vi "set_refdac.vi"(0 "TSM context":T2, 5 "Config PVS":T1 {"VREFN" format="%#_13g"; "AVOUT" format="%#_13g"; "VREFP" format="%#_13g"; "Read/Write" items=["Write", "Read"]}, 11 "Error In":errorcluster) -> (4 "TSM context Out":T2, 15 "Error Out":errorcluster)   [LabVIEW 2019]
doc: "This VI set the output voltage of Precision Voltage Source (PVS)"
uses:
  <vilib>/NI_TestStand_SemiconductorModule/NI_TestStand_Semiconductor_Module.lvlibp/PinMap/General/SemiconductorModuleContext.ctl
  typedefs/set_refdac_param.ctl
  <instrlib>/niDigital/niDigital.llb/niDigital Selected Function.ctl
  <instrlib>/niDigital/niDigital.llb/niDigital Write Static Pin State.ctl
  <instrlib>/niDigital/niDigital.llb/niDigital Data Mapping.ctl
  <instrlib>/niDigital/niDigital.llb/niDigital Bit Order.ctl
  Instrument Control/Digital/SSC Digital/Configuration/SSC Digital Select Function.vi
  Instrument Control/Digital/SSC Digital/Static/SSC Digital Write Static.vi
  <instrlib>/niDigital/niDigital.llb/niDigital Create Source Waveform (Serial).vi
  <instrlib>/niDigital/niDigital.llb/niDigital Write Source Waveform (Broadcast U32).vi
  <instrlib>/niDigital/niDigital.llb/niDigital Burst Pattern (Pass Fail).vi
  <vilib>/NI_TestStand_SemiconductorModule/NI_TestStand_Semiconductor_Module.lvlibp/PinMap/Digital Pattern/PinsToNIDigitalPatternSessions.vi
  <vilib>/NI_TestStand_SemiconductorModule/NI_TestStand_Semiconductor_Module.lvlibp
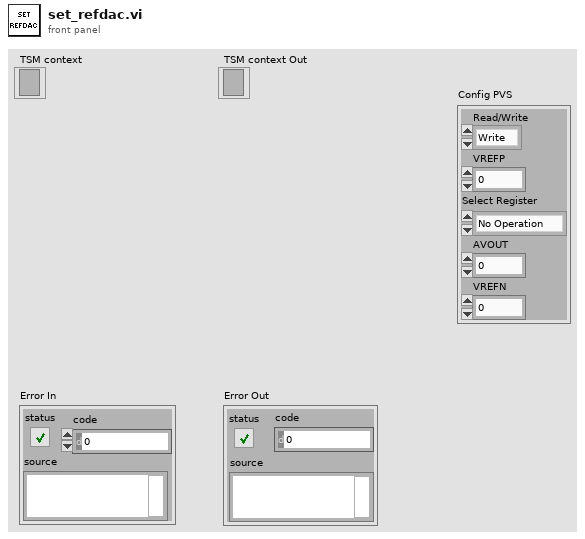
[diagram p1: front panel]
types:
  T1 = typedef "set_refdac_param.ctl" = cluster{"Read/Write":u16, "VREFP":dbl, "Select Register":enum16{"No Operation", "DAC Register", "Control Register", "Clearcode Register", "Software Control Register"}, "AVOUT ":dbl, "VREFN":dbl}
  T2 = typedef "NI_TestStand_Semiconductor_Module.lvlibp/SemiconductorModuleContext.ctl" = refnum<k7>
  T3 = enum16{"No Operation", "DAC Register", "Control Register", "Clearcode Register", "Software Control Register"}
  T4 = typedef "niDigital Bit Order.ctl" = i32
  T5 = typedef "niDigital Data Mapping.ctl" = i32
  T6 = typedef "niDigital Write Static Pin State.ctl" = u8
  T7 = typedef "niDigital Selected Function.ctl" = i32
  T8 = typedef "TSM SSC Digital.ctl" = cluster{"Pin Query Context":refnum<class "DigitalPatternPinQueryContext.lvclass">, "SSC":T9[], "Site Numbers":i32[], "Pins":tag[]}
  T9 = typedef "SSC Digital.ctl" = cluster{"Session":refnum<k15>, "Channel List":string, "Site List":string}
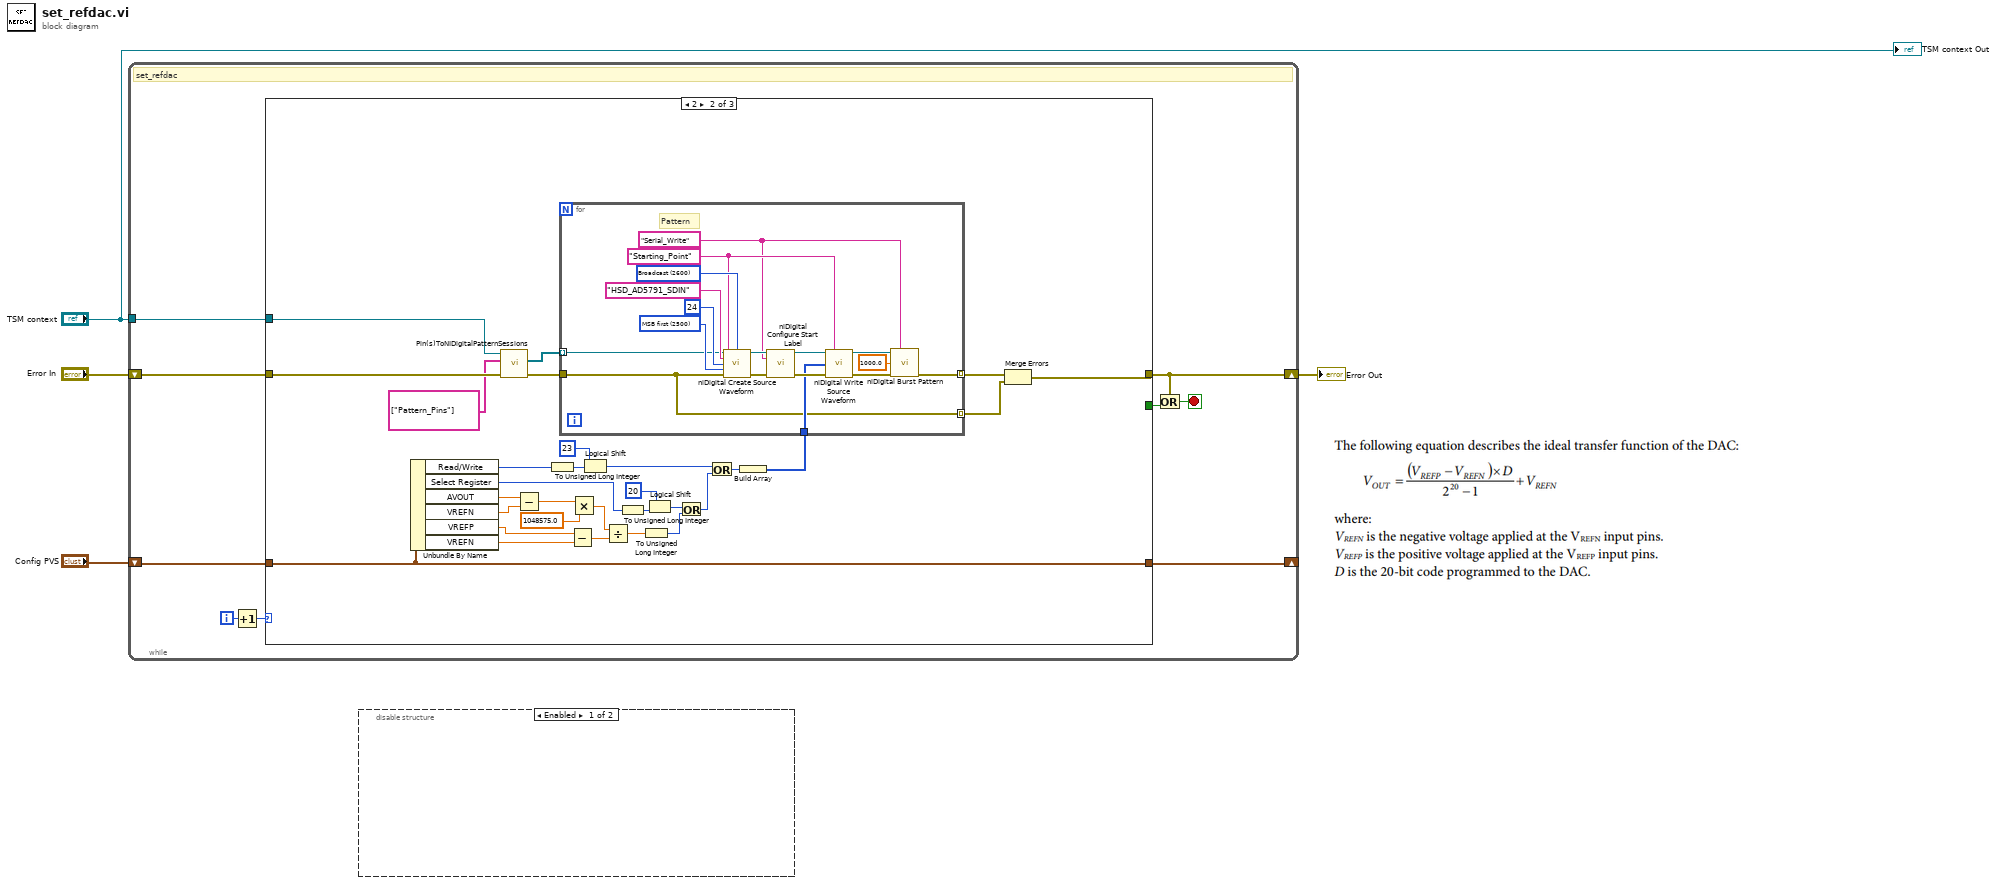
[diagram p0: block diagram]
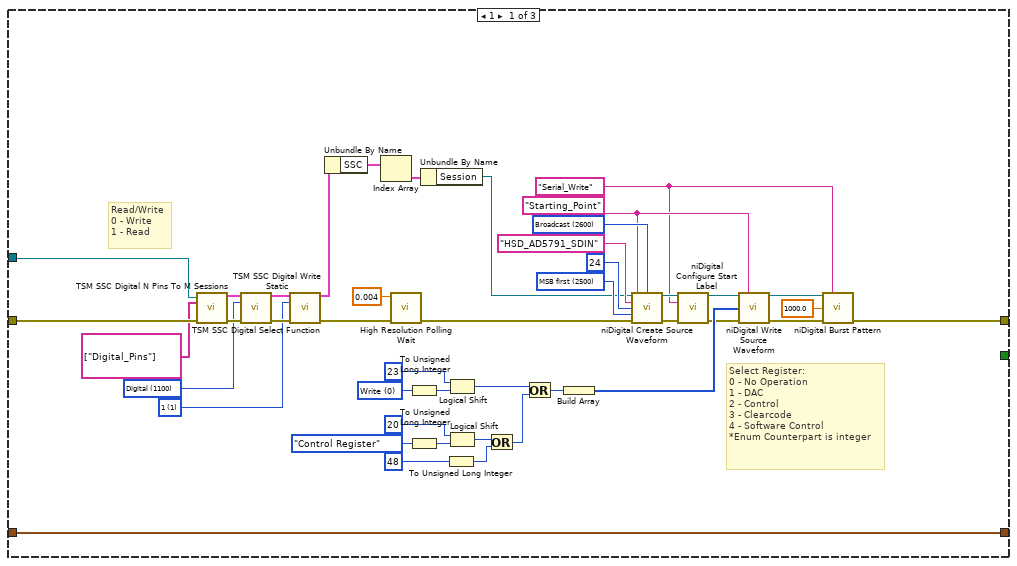
[diagram p3: hidden frame]
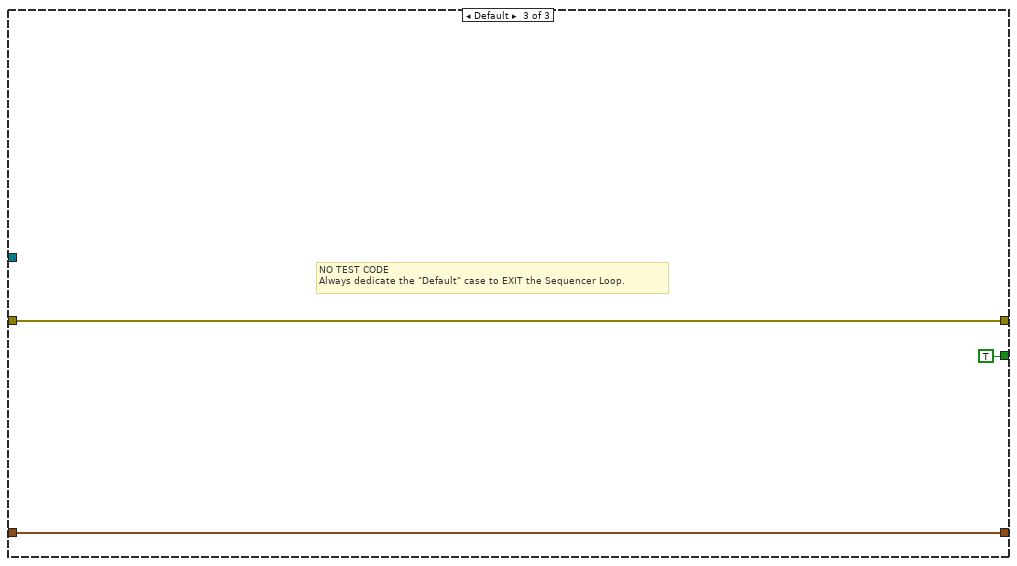
[diagram p4: hidden frame]
diagram:
  n1 = while {
    shift-right: [w7] -> w2
    shift-left: "Error In" -> [w12]
    tunnel: "TSM context" -> [w10]
    shift-right: [w6] -> _
    shift-left: "Config PVS" -> [w5]
    i -> [w13]
    stop <- w8 stop-if-true
    # "set_refdac"
    n2 = Increment(x=w13) -> (x+1=w11:i32)
    n3 = case shown="2" w11 {
      tunnel: [w16 w66 w106] -> w7
      tunnel: w12 -> [w42 w86 w106]
      tunnel: w10 -> [w40 w87 _]
      tunnel: [_ _ TRUE] -> w9
      tunnel: [w45 w69 w105] -> w6
      tunnel: w5 -> [w45 w69 w105]
      frame 1 {
        w29 = T4 2500 items=["MSB first"=2500, "LSB first"=2501] ("bit order")
        w31 = T5 2600 items=["Broadcast"=2600, "Site Unique"=2601] ("data mapping")
        w22 = "Serial_Write" ("Pattern")
        w26 = "Starting_Point" ("waveform name")
        w33 = T6 1 items=["0"=0, "1"=1, "X"=5] ("State")
        w35 = T7 1100 items=["Digital"=1100, "PPMU"=1101, "Off"=1102, "Disconnect"=1103] ("Function")
        w50 = u16 0 items=["Write", "Read"] ("Read/Write 2")
        # "Read/Write\n0 - Write\n1 - Read"
        # "Select Register:\n0 - No Operation\n1 - DAC\n2 - Control\n3 - Clearcode\n4 - Software Control\n*Enum Counterpart is integer"
        n4 = call "TSM SSC Digital N Pins To M Sessions.vi"("TSM context"=w40, "Pins"=tag[] ["Digital_Pins"], "error in"=w42) -> ("Digital TSM Out"=w38:T8, "error out"=w41:errorcluster)  [unwired: 11 in]
        n5 = call "TSM SSC Digital Select Function.vi"("Digital TSM In"=w38, "Function"=w35, "error in"=w41) -> ("Digital TSM Out"=w36:T8, "error out"=w34:errorcluster)  [unwired: 11 in]
        n6 = call "TSM SSC Digital Write Static.vi"("Digital TSM in"=w36, "State"=w33, "error in"=w34) -> ("Digital TSM out"=w17:T8, "error out"=w37:errorcluster)  [unwired: 11 in]
        n7 = Unbundle By Name(w17) -> ("SSC"=w20:T9[])
        n8 = Index Array(array=w20) -> (element=w19:T9)  [unwired: 1 in]
        n9 = call <vilib>:"High Resolution Polling Wait.vi"("error in (no error)"=w37, "seconds to wait"=0.004) -> ("error out"=w44:errorcluster)  [unwired: 9 in]
        n10 = To Unsigned Long Integer(number=w50) -> (unsigned 32bit integer=w49:u32)
        n11 = To Unsigned Long Integer(number=T3."Control Register" ("Select Register 2")) -> (unsigned 32bit integer=w46:u32)
        n12 = Unbundle By Name(w19) -> ("Session"=w18:refnum<k15>)
        n13 = To Unsigned Long Integer(number=48 ("Data To Write")) -> (unsigned 32bit integer=w47:u32)
        n14 = Logical Shift(y=u16 23 ("x"), x=w49) -> (x << y=w54:u32)
        n15 = Logical Shift(y=i16 20, x=w46) -> (x << y=w53:u32)
        n16 = Or(x=w53, y=w47) -> (x .or. y?=w52:u32)
        n17 = Or(x=w54, y=w52) -> (x .or. y?=w57:u32)
        n18 = Build Array(w57) -> (w55:u32[])
        n19 = call-poly <instrlib>:"niDigital Create Source Waveform.vi"("instrument handle"=w18, "waveform name"=w26, "data mapping"=w31, "pin list"="HSD_AD5791_SDIN", "sample width"=u32 24, "bit order"=w29, "error in"=w44) -> ("instrument handle out"=w32:refnum<k15>, "error out"=w23:errorcluster)  [unwired: 7 in]
        n20 = call <instrlib>:"niDigital Configure Start Label.vi"("instrument handle"=w32, "start label"=w22, "error in"=w23) -> ("instrument handle out"=w28:refnum<k15>, "error out"=w27:errorcluster)  [unwired: 11 in]
        n21 = call-poly <instrlib>:"niDigital Write Source Waveform.vi"("instrument handle"=w28, "waveform name"=w26, "waveform data"=w55, "error in"=w27) -> ("instrument handle out"=w25:refnum<k15>, "error out"=w24:errorcluster)  [unwired: 10 in]
        n22 = call-poly <instrlib>:"niDigital Burst Pattern.vi"("instrument handle"=w25, "start label"=w22, "timeout (s)"=1000.0, "error in"=w24) -> ("error out"=w16:errorcluster)  [unwired: 9 in, 2 out]
      }
      frame 2 {
        n23 = Unbundle By Name(w69) -> ("Read/Write"=w65:u16, "Select Register"=w64:T3, "AVOUT"=w63:dbl, "VREFN"=w62:dbl, "VREFP"=w60:dbl, "VREFN"=w59:dbl)
        n24 = call-poly <vilib>:"Pin(s)ToNIDigitalPatternSessions.vi"("error in (no error)"=w86, "Pins"=tag[] ["Pattern_Pins"], "Semiconductor Module Context"=w87) -> ("error out"=w83:errorcluster, "Instrument Sessions"=w84:refnum<k15>[])  [unwired: 3 in, 4 out]
        n25 = Subtract(x=w63, y=w62) -> (x-y=w61:dbl)
        n26 = To Unsigned Long Integer(number=w65) -> (unsigned 32bit integer=w72:u32)
        n27 = Subtract(x=w60, y=w59) -> (x-y=w58:dbl)
        n28 = Multiply(x=w61, y=1048575.0) -> (x*y=w74:dbl)
        n29 = Logical Shift(y=u16 23 ("x"), x=w72) -> (x << y=w80:u32)
        n30 = Divide(x=w74, y=w58) -> (x/y=w76:dbl)
        n31 = To Unsigned Long Integer(number=w64) -> (unsigned 32bit integer=w71:u32)
        n32 = To Unsigned Long Integer(number=w76) -> (unsigned 32bit integer=w70:u32)
        n33 = Logical Shift(y=i16 20, x=w71) -> (x << y=w79:u32)
        n34 = Or(x=w79, y=w70) -> (x .or. y?=w78:u32)
        n35 = Or(x=w80, y=w78) -> (x .or. y?=w82:u32)
        n36 = Build Array(w82) -> (w73:u32[])
        n37 = for {
          tunnel: w83 -> [w89]
          tunnel: w84 -> [w96] mode=indexing
          tunnel: [w94] -> w68 mode=indexing
          tunnel: w73 -> [w90]
          tunnel: [w89] -> w67 mode=indexing
          w101 = T4 2500 items=["MSB first"=2500, "LSB first"=2501] ("bit order")
          w103 = T5 2600 items=["Broadcast"=2600, "Site Unique"=2601] ("data mapping")
          w91 = "Serial_Write" ("Pattern")
          w97 = "Starting_Point" ("waveform name")
          # "Pattern"
          n38 = call-poly <instrlib>:"niDigital Create Source Waveform.vi"("instrument handle"=w96, "waveform name"=w97, "data mapping"=w103, "pin list"="HSD_AD5791_SDIN", "sample width"=u32 24, "bit order"=w101, "error in"=w89) -> ("instrument handle out"=w104:refnum<k15>, "error out"=w95:errorcluster)  [unwired: 7 in]
          n39 = call <instrlib>:"niDigital Configure Start Label.vi"("instrument handle"=w104, "start label"=w91, "error in"=w95) -> ("instrument handle out"=w100:refnum<k15>, "error out"=w98:errorcluster)  [unwired: 11 in]
          n40 = call-poly <instrlib>:"niDigital Write Source Waveform.vi"("instrument handle"=w100, "waveform name"=w97, "waveform data"=w90, "error in"=w98) -> ("instrument handle out"=w92:refnum<k15>, "error out"=w93:errorcluster)  [unwired: 10 in]
          n41 = call-poly <instrlib>:"niDigital Burst Pattern.vi"("instrument handle"=w92, "start label"=w91, "timeout (s)"=1000.0, "error in"=w93) -> ("error out"=w94:errorcluster)  [unwired: 9 in, 2 out]
        }
        n42 = Merge Errors(w68, w67) -> (w66:errorcluster)
      }
      frame Default {
        # "NO TEST CODE\nAlways dedicate the \"Default\" case to EXIT the Sequencer Loop."
        # "Exit Loop"
      }
    }
    n43 = Or(x=w7, y=w9) -> (x .or. y?=w8:bool)
  }
  "Error Out" <- w2
  n44 = disable-structure shown="Enabled" {
    frame Enabled {
    }
    frame Disabled {
    }
  }
  "TSM context Out" <- "TSM context"
